vi "nanocal -- nuclear schottky fit V4.vi"() -> ()   [LabVIEW 2020] (continued)
  w19 = string[] ["T", "B", "theta", "side", "zeta", "tau1", "tauS", "tauN", "tauC", "kappa0"]  # names in latin
  w17 = string[] ["T", "B", "θ", "side", "ζ", "τ1", "τS", "τN", "τC", "κ0"]  # names greek
  w21 = map{T5, map{T11, string}} {}  # Size: 0
  w20 = T5[] [enum."T (K)", enum."B (T)", enum."θ (deg)", enum."side (S|R)", enum."ζ", enum."τ1", enum."τS", enum."τN", enum."τC", enum."κ0"] items=["ζ", "τ1", "τS", "τN", "τC", "κ0", "m1", "m2", "m3", "T (K)", "B (T)", "θ (deg)", "side (S|R)", "change (B|T)"]
  w27 = dbl[] []
  (unwired) u32[] [10967551, 1239551, 2785279, 16734592, 16755712, 8795, 8285330, 9272482, 9204890]
  w23 = T5[] [enum."ζ", enum."τ1", enum."τS", enum."τN", enum."τC", enum."κ0"] items=["ζ", "τ1", "τS", "τN", "τC", "κ0", "m1", "m2", "m3", "T (K)", "B (T)", "θ (deg)", "side (S|R)", "change (B|T)"]
  w33 = map{T5, i32} {}  # Size: 0
  w28 = T5[] [enum."ζ", enum."τ1", enum."τS", enum."τN", enum."τC", enum."κ0", enum."m1", enum."m2", enum."m3"] items=["ζ", "τ1", "τS", "τN", "τC", "κ0", "m1", "m2", "m3", "T (K)", "B (T)", "θ (deg)", "side (S|R)", "change (B|T)"]
  w34 = FALSE ("newton pause")
  w36 = map{T5, dbl} {}  # Size: 0
  w37 = 0.0 ("new X")
  w51 = "void"  # interface
  w53 = "void"  # action
  # "init file meta semantics -- external (file) part of the file key"
  # "cursor indices and plot colors"
  # "selector name semantics"
  # "init side semantics -- internal part of the file key"
  n1 = for {
    shift-right: [w62] -> w10
    shift-left: w13 -> [w63]
    tunnel: string[] ["_ref_", "_sam_"] -> [w59] mode=indexing
    tunnel: i32[] [4000, 8000] -> [w56] mode=indexing
    tunnel: w9 -> [w55] mode=indexing
    shift-right: [w60] -> w7
    shift-left: w8 -> [w61]
    shift-right: [w57] -> w5
    shift-left: w6 -> [w58]
    n2 = Insert Into Map(map in=w58, key=w56, value=w55) -> (map out=w57:map{i32, T14})  [unwired: 2 out]
    n3 = Insert Into Map(map in=w61, key=w55, value=w59) -> (map out=w60:map{T14, string})  [unwired: 2 out]
    n4 = Insert Into Map(map in=w63, key=w55, value=w56) -> (map out=w62:map{T14, i32})  [unwired: 2 out]
  }
  "side map from NUM" <- w5
  "side map to STR" <- w7
  "side map to NUM" <- w10
  n5 = for {
    shift-right: [w66] -> w4
    shift-left: w3 -> [w67]
    tunnel: w2 -> [w65] mode=indexing
    tunnel: w1 -> [w64] mode=indexing
    n6 = Insert Into Map(map in=w67, key=w65, value=w64) -> (map out=w66:map{T5, T15})  [unwired: 2 out]
  }
  "data file parameters map" <- w4
  n7 = for {
    shift-right: [w70] -> w31
    shift-left: w33 -> [w71]
    tunnel: w28 -> [w69] mode=indexing
    tunnel: i32[] [0, 1, 2, 3, 4, 5, 6, 7, 8] -> [w68] mode=indexing
    n8 = Insert Into Map(map in=w71, key=w69, value=w68) -> (map out=w70:map{T5, i32})  [unwired: 2 out]
  }
  n9 = for {
    shift-right: [w86] -> w15
    shift-left: w21 -> [w87]
    tunnel: w19 -> [w77] mode=indexing
    tunnel: w20 -> [w85] mode=indexing
    tunnel: w18 -> [w75]
    tunnel: w17 -> [w76] mode=indexing
    tunnel: w16 -> [w78] mode=indexing
    tunnel: w14 -> [w74] mode=indexing
    n10 = Insert Into Map(map in=w75, key=nameformattingitem."prec", value=w74) -> (map out=w73:map{T11, string})  [unwired: 2 out]
    n11 = Insert Into Map(map in=w73, key=nameformattingitem."name", value=w76) -> (map out=w84:map{T11, string})  [unwired: 2 out]
    n12 = Insert Into Map(map in=w84, key=nameformattingitem."nameL" ("name formatting item"), value=w77) -> (map out=w83:map{T11, string})  [unwired: 2 out]
    n13 = Insert Into Map(map in=w83, key=nameformattingitem."units" ("name formatting item"), value=w78) -> (map out=w82:map{T11, string})  [unwired: 2 out]
    n14 = Insert Into Map(map in=w87, key=w85, value=w82) -> (map out=w86:map{T5, map{T11, string}})  [unwired: 2 out]
  }
  "new selector names" <- w15
  n15 = local write "cursor index map"(w31) -> ()
  n16 = local write "newton action"(3-lorentzian-heat-response_action."onlygrads" ("newton action")) -> ()
  n17 = Bundle(w27, w27) -> (w26:cluster{dbl[], dbl[]})  [unwired: 1 in]
  n18 = Initialize Array(w26, 5 ("dimension size")) -> (→"Plot: goodness vs parameter":cluster{dbl[], dbl[]}[])
  n19 = control-ref of="Plot: sweep window"() -> (w43:refnum<vi>)
  n20 = Bundle By Name(cluster=T2 {"left"=0.0, "right "=0.0, "center"=0.0, "window"=0.0, "cursors"=[], "relative"=0, "absolute"=0, "fixed vertical offset"=0.0, "vertical offset"=0.0, "skew"=0.0, "default window frac"=0.0, "kind"=enum."symmetric", "skew.left"=0.0, "skew.right"=0.0, "Plot ref"=refnum, "wing order"=enum."forw"} ("cursor bracket: All, data window"), "Plot ref"=w43, "cursors"=i32[] [0, 1, 2], "fixed vertical offset"=0.0, "default window frac"=0.3 ("fixed vertical offset"), "kind"=enum16{"symmetric", "skewed", "fancy"}."symmetric") -> (w46:T2)
  n21 = local write "what"(cluster{"scaling":dbl, "what":T5}[] [{"scaling"=1.0, "what"=enum."ζ"}, {"scaling"=1.0, "what"=enum."τ1"}, {"scaling"=1.0, "what"=enum."τS"}, {"scaling"=1.0, "what"=enum."τN"}, {"scaling"=1.0, "what"=enum."τC"}, {"scaling"=1.0, "what"=enum."κ0"}]) -> ()
  n22 = control-ref of="cursor window"() -> (w42:refnum<vi>)
  n23 = Create User Event(user event datatype=w53) -> (user event=w41:refnum<user-event>)  [unwired: 1 in, 1 out]
  n24 = call "cursor window logic V3.vi"("cursor window action"=cursor_window_action."init", "cursor window in"=w42, "cursor window init"=w46) -> ()  [unwired: 7 in, 2 out]
  n25 = register-events(w41) -> (reference out=w54:refnum<event-registration>)  [unwired: 2 in, 1 out]
  n26 = Create User Event(user event datatype=w51) -> (user event=w29:refnum<user-event>)  [unwired: 1 in, 1 out]
  n27 = local write "parameter"(w23) -> ()
  n28 = register-events(w29) -> (reference out=w52:refnum<event-registration>)  [unwired: 2 in, 1 out]
  n29 = control-ref of="Plot: sweep window"() -> (w38:refnum<vi>)
  n30 = while "actions" {
    tunnel: w54 -> [w92]
    tunnel: w41 -> [w91]
    tunnel: w29 -> [w89]
    tunnel: w23 -> [w88]
    stop <- w90 stop-if-true
    n31 = event shown="[0] <action>: User Event" {
      selector: w92 -> [_]
      dyn-events: _ -> [_]
      timeout: _ -> [_]
      tunnel: w91 -> [w96]
      tunnel: [w95] -> w90
      tunnel: w89 -> [w94]
      tunnel: w88 -> [w93]
      event User Event {
        n32 = event-data() -> ("action"=w97:string)  [unwired: 1 in]
        n33 = case shown="\"action: constrained filenames select\"" w97 {
          tunnel: w96 -> [w98 _ _ w350 w457 w475 w495 _ w651 _ w769 _ _ w904 _ w981 w1020 _ w1077 _ _]
          tunnel: [_ _ _ _ _ _ _ _ _ _ _ _ _ _ _ _ _ TRUE _ _ _] -> w95
          tunnel: w94 -> [_ _ _ w349 _ _ _ _ _ _ _ _ _ _ _ _ _ _ _ _ _]
          tunnel: w93 -> [w100 w177 w233 _ _ _ _ _ _ _ _ _ w816 _ _ _ _ _ _ _ _]
          frame "action: new sweep" {
            (unwired) 3-lorentzian-heat-response_action."onlygrads" ("action")
            w106 = T5[] [enum."m1", enum."m2", enum."m3"] items=["ζ", "τ1", "τS", "τN", "τC", "κ0", "m1", "m2", "m3", "T (K)", "B (T)", "θ (deg)", "side (S|R)", "change (B|T)"]
            w112 = T5[] [enum."T (K)", enum."B (T)", enum."θ (deg)"] items=["ζ", "τ1", "τS", "τN", "τC", "κ0", "m1", "m2", "m3", "T (K)", "B (T)", "θ (deg)", "side (S|R)", "change (B|T)"]
            w149 = 6.283185307179586
            n34 = Generate User Event(user event=w98, event data cluster="action: reset colors" ("event data")) -> ()  [unwired: 2 in, 2 out]
            n35 = local read "T1"() -> (w135:dbl)
            n36 = call "nanocal -- publish -- freq scan V2.vi"("publisher action"=publisher_action."get") -> ("dz/dω out (V)"=w150:cdb[], "z out (V)"=w145:cdb[], "ω out (Hz)"=w152:dbl[])  [unwired: 8 in]
            n37 = local read "τS"() -> (w134:dbl)
            n38 = local read "τN"() -> (w133:dbl)
            n39 = local read "τC"() -> (w132:dbl)
            n40 = local read "κ0"() -> (w131:dbl)
            n41 = local read "ζ"() -> (w136:dbl)
            n42 = Divide(x=w150, y=w149) -> (x/y=w147:cdb[])
            n43 = Multiply(x=w152, y=w149) -> (x*y=w144:dbl[])
            n44 = Build Array (concatenate)(w100, w106) -> (w105:T5[])
            n45 = Build Array(w136, w135, w134, w133, w132, w131) -> (w118:dbl[])
            n46 = local read "newton action"() -> (w101:T9)
            n47 = for {
              shift-right: [w163] -> w104
              shift-left: map{T5, dbl} {} ("Map IN") -> [w164]
              tunnel: w105 -> [w161] mode=indexing
              tunnel: w118 -> [w162] mode=indexing
              tunnel: [w161] -> w107 mode=indexing
              n48 = Insert Into Map(map in=w164, key=w161, value=w162) -> (map out=w163:map{T5, dbl})  [unwired: 2 out]
            }
            n49 = local read "weighting"() -> (w146:T8)
            n50 = call "nanocal -- nuclear schottky goodness V5.vi"("action"=w101, "parameters IN"=w104, "weighting strategy"=w146, "dz/dω IN (V)"=w147, "Voltage IN (V)"=w145, "ω (rad/sec)"=w144) -> ("R norm"=w143:dbl, "G"=w142:dbl, "R(ω) out"=w141:cdb[], "dG / d log α   OUT"=w103:map{T5, dbl})  [unwired: 2 in]
            n51 = for {
              tunnel: w100 -> [w155] mode=indexing
              shift-right: [w156] -> _
              shift-left: w103 -> [w156]
              tunnel: [w154] -> w102 mode=indexing
              n52 = Look In Map(map=w156, key=w155) -> (value=w154:dbl)  [unwired: 1 in, 1 out]
            }
            "logarithmic derivatives" <- w102
            n53 = Divide(x=w142, y=w143) -> (x/y=→"goodness":dbl)
            n54 = local read "θ (deg)"() -> (w114:dbl)
            n55 = local read "B (T)"() -> (w115:dbl)
            n56 = local read "T (K)"() -> (w116:dbl)
            n57 = call "3-lorentzian-heat-response -- V4.vi"("action"=3-lorentzian-heat-response_action."calc m1m2m3", "Map IN"=w104) -> ("Map OUT"=w113:map{T5, dbl})  [unwired: 7 in, 2 out]
            n58 = Build Array(w116, w115, w114) -> (w111:dbl[])
            n59 = local read "cursor x selector"() -> (w140:map{T5, dbl})
            n60 = local read "X selector"() -> (w139:T5)
            n61 = local read "cursor index map"() -> (w120:map{T5, i32})
            n62 = for {
              shift-right: [w159] -> w110
              shift-left: w113 -> [w160]
              tunnel: w112 -> [w158] mode=indexing
              tunnel: w111 -> [w157] mode=indexing
              n63 = Insert Into Map(map in=w160, key=w158, value=w157) -> (map out=w159:map{T5, dbl})  [unwired: 2 out]
            }
            n64 = local read "T (K)"() -> (w138:dbl)
            n65 = control-ref of="Plot:  colors"() -> (w151:refnum<vi>)
            n66 = control-ref of="Plot: sweep window"() -> (w130:refnum<vi>)
            n67 = Complex To Re/Im(x + iy=w145) -> (x=w129:dbl[], y=w128:dbl[])
            n68 = Look In Map(map=w140, key=w139, default value=w138) -> (value=w137:dbl)  [unwired: 1 out]
            n69 = call "replace plot - plot ref - V2.vi"("Plot ref in"=w130, "Array X IN"=w129, "Array Y IN"=w128, "plot index"=enum16{"data R(ω)", "fit R(ω)"}."data R(ω)" ("Plost: sweep window"), "cursor action"=cursor_action."write") -> ("Plot ref out"=w127:refnum<vi>)  [unwired: 11 in, 3 out]
            n70 = for {
              tunnel: w137 -> [w172]
              tunnel: w151 -> [w171]
              tunnel: w107 -> [w167] mode=indexing
              tunnel: w120 -> [w169]
              shift-right: [w166] -> _
              shift-left: w113 -> [w166]
              n71 = Look In Map(map=w166, key=w167) -> (value=w165:dbl)  [unwired: 1 in, 1 out]
              n72 = Look In Map(map=w169, key=w167) -> (value=w168:i32)  [unwired: 1 in, 1 out]
              n73 = call "replace cursor - plot ref - V2.vi"("Plot ref in"=w171, "new X"=w172, "new  Y"=w165, "cursor index"=w168, "cursor action"=cursor_action."write") -> ()  [unwired: 11 in, 4 out]
            }
            n74 = call "string parse mathematica assosiated array.vi"("derivative"=mathematica_string_map_action."create string", "Map IN"=w110) -> ("String OUT"=w108:string)  [unwired: 8 in, 1 out]
            n75 = Complex To Re/Im(x + iy=w141) -> (x=w125:dbl[], y=w124:dbl[])
            n76 = local write "String"(w108) -> ()
            n77 = call "replace plot - plot ref - V2.vi"("Plot ref in"=w127, "Array X IN"=w125, "Array Y IN"=w124, "plot index"=enum16{"data R(ω)", "fit R(ω)"}."fit R(ω)" ("Plost: sweep window"), "cursor action"=cursor_action."write") -> ()  [unwired: 11 in, 4 out]
          }
          frame "action: replot circles" {
            w205 = 6.283185307179586
            n78 = call "nanocal -- publish -- freq scan V2.vi"("publisher action"=publisher_action."get") -> ("dz/dω out (V)"=w206:cdb[], "z out (V)"=w202:cdb[], "ω out (Hz)"=w207:dbl[])  [unwired: 8 in]
            n79 = local read "T1"() -> (w196:dbl)
            n80 = local read "τS"() -> (w195:dbl)
            n81 = local read "κ0"() -> (w192:dbl)
            n82 = local read "τN"() -> (w194:dbl)
            n83 = local read "τC"() -> (w193:dbl)
            n84 = local read "ζ"() -> (w197:dbl)
            n85 = Divide(x=w206, y=w205) -> (x/y=w204:cdb[])
            n86 = Multiply(x=w207, y=w205) -> (x*y=w201:dbl[])
            n87 = Build Array(w197, w196, w195, w194, w193, w192) -> (w178:dbl[])
            n88 = for {
              shift-right: [w214] -> w176
              shift-left: map{T5, dbl} {} ("Map IN") -> [w215]
              tunnel: w177 -> [w213] mode=indexing
              tunnel: [w212] -> _ mode=indexing
              tunnel: [w213] -> w174 mode=indexing
              tunnel: w178 -> [w212] mode=indexing
              n89 = Insert Into Map(map in=w215, key=w213, value=w212) -> (map out=w214:map{T5, dbl})  [unwired: 2 out]
            }
            n90 = local read "weighting"() -> (w203:T8)
            n91 = call "nanocal -- nuclear schottky goodness V5.vi"("action"=3-lorentzian-heat-response_action."onlygrads", "parameters IN"=w176, "weighting strategy"=w203, "dz/dω IN (V)"=w204, "Voltage IN (V)"=w202, "ω (rad/sec)"=w201) -> ("R norm"=w200:dbl, "G"=w199:dbl, "R(ω) out"=w198:cdb[], "dG / d log α   OUT"=w175:map{T5, dbl})  [unwired: 2 in]
            n92 = control-ref of="Plot: sweep window"() -> (w188:refnum<vi>)
            n93 = Divide(x=w199, y=w200) -> (x/y=w191:dbl)
            n94 = for {
              tunnel: w174 -> [w210] mode=indexing
              shift-right: [w211] -> _
              shift-left: w175 -> [w211]
              tunnel: [w209] -> w173 mode=indexing
              n95 = Look In Map(map=w211, key=w210) -> (value=w209:dbl)  [unwired: 1 in, 1 out]
            }
            n96 = Complex To Re/Im(x + iy=w202) -> (x=w186:dbl[], y=w185:dbl[])
            n97 = local write "goodness"(w191) -> ()
            n98 = call "replace plot - plot ref - V2.vi"("Plot ref in"=w188, "Array X IN"=w186, "Array Y IN"=w185, "plot index"=enum16{"data R(ω)", "fit R(ω)"}."data R(ω)" ("Plost: sweep window"), "cursor action"=cursor_action."write") -> ("Plot ref out"=w187:refnum<vi>)  [unwired: 11 in, 3 out]
            n99 = Complex To Re/Im(x + iy=w198) -> (x=w184:dbl[], y=w183:dbl[])
            n100 = local write "logarithmic derivatives"(w173) -> ()
            n101 = call "replace plot - plot ref - V2.vi"("Plot ref in"=w187, "Array X IN"=w184, "Array Y IN"=w183, "plot index"=enum16{"data R(ω)", "fit R(ω)"}."fit R(ω)" ("Plost: sweep window"), "cursor action"=cursor_action."write") -> ()  [unwired: 11 in, 4 out]
          }
          frame "action: plot landscape" {
            w225 = array_action."generate log range" ("action")
            w247 = 6.283185307179586
            n102 = property on="range one" class="Slide (strict)"() -> ("Scale.Range"=w237:T29)  [unwired: 2 in, 2 out]
            n103 = property on="range two" class="Slide (strict)"() -> ("Scale.Range"=w236:T29)  [unwired: 2 in, 2 out]
            n104 = Unbundle By Name(w237) -> ("Maximum"=w228:dbl, "Minimum"=w227:dbl)
            n105 = Unbundle By Name(w236) -> ("Maximum"=w230:dbl, "Minimum"=w229:dbl)
            n106 = local read "ζ"() -> (w243:dbl)
            n107 = local read "T1"() -> (w242:dbl)
            n108 = local read "τS"() -> (w241:dbl)
            n109 = local read "τN"() -> (w240:dbl)
            n110 = local read "τC"() -> (w239:dbl)
            n111 = local read "κ0"() -> (w238:dbl)
            n112 = call "nanocal -- publish -- freq scan V2.vi"("publisher action"=publisher_action."get") -> ("dz/dω out (V)"=w248:cdb[], "z out (V)"=w245:cdb[], "ω out (Hz)"=w249:dbl[])  [unwired: 8 in]
            n113 = local read "cursor index map"() -> (w219:map{T5, i32})
            n114 = Build Array(w243, w242, w241, w240, w239, w238) -> (w224:dbl[])
            n115 = call "array -- generate range -- V5.vi"("action"=w225, "ω points"="# points", "ω from"=w227, "ω to"=w228) -> ("ω out"=w226:dbl[])  [unwired: 7 in]
            n116 = call "array -- generate range -- V5.vi"("action"=w225, "ω points"="# points", "ω from"=w229, "ω to"=w230) -> ("ω out"=w231:dbl[])  [unwired: 7 in]
            n117 = local read "color Map"() -> (w220:map{T5, u32})
            n118 = Divide(x=w248, y=w247) -> (x/y=w246:cdb[])
            n119 = Multiply(x=w249, y=w247) -> (x*y=w244:dbl[])
            n120 = for {
              shift-right: [w340] -> w232
              shift-left: map{T5, dbl} {} ("Map IN") -> [w341]
              tunnel: w233 -> [w339] mode=indexing
              tunnel: w224 -> [w338] mode=indexing
              n121 = Insert Into Map(map in=w341, key=w339, value=w338) -> (map out=w340:map{T5, dbl})  [unwired: 2 out]
            }
            n122 = Look In Map(map=w220, key="two") -> (value=w222:u32)  [unwired: 1 in, 1 out]
            n123 = Look In Map(map=w220, key="one") -> (value=w221:u32)  [unwired: 1 in, 1 out]
            n124 = property on="range one" class="Slide (strict)"("Fill Color"=w221) -> ()  [unwired: 2 in, 2 out]
            n125 = Build Array("one", "two") -> (w218:T5[])
            n126 = property on="range two" class="Slide (strict)"("Fill Color"=w222) -> ()  [unwired: 2 in, 2 out]
            n127 = case shown="\"2d plots \"" "what" {
              tunnel: w246 -> [w259 w302]
              tunnel: w245 -> [w258 w301]
              tunnel: w244 -> [w257 w300]
              tunnel: w232 -> [w256 w299]
              tunnel: "one" -> [_ w298]
              tunnel: w231 -> [_ w297]
              tunnel: w226 -> [w255 w296]
              tunnel: "two" -> [_ w295]
              tunnel: w220 -> [w254 _]
              tunnel: w219 -> [w253 _]
              tunnel: w218 -> [w251 _]
              frame "1d plots", Default {
                n128 = control-ref of="Plot: goodness vs parameter"() -> (w252:refnum<vi>)
                n129 = for {
                  tunnel: w259 -> [w278]
                  tunnel: w258 -> [w277]
                  tunnel: w257 -> [w276]
                  tunnel: w256 -> [w263]
                  tunnel: w255 -> [w272]
                  tunnel: w251 -> [w262] mode=indexing
                  tunnel: w254 -> [w269]
                  tunnel: w253 -> [w268]
                  tunnel: w252 -> [w260]
                  n130 = for {
                    tunnel: w278 -> [w283]
                    tunnel: w277 -> [w285]
                    tunnel: w276 -> [w284]
                    tunnel: w272 -> [w280] mode=indexing
                    tunnel: [w288] -> w274 mode=indexing
                    tunnel: [w280] -> w273 mode=indexing
                    tunnel: w263 -> [w281]
                    tunnel: w262 -> [w282]
                    n131 = Insert Into Map(map in=w281, key=w282, value=w280) -> (map out=w279:map{T5, dbl})  [unwired: 2 out]
                    n132 = local read "weighting"() -> (w287:T8)
                    n133 = call "nanocal -- nuclear schottky goodness V5.vi"("action"=3-lorentzian-heat-response_action."onlygrads", "parameters IN"=w279, "weighting strategy"=w287, "dz/dω IN (V)"=w283, "Voltage IN (V)"=w285, "ω (rad/sec)"=w284) -> ("R norm"=w290:dbl, "G"=w289:dbl)  [unwired: 2 in, 2 out]
                    n134 = Divide(x=w289, y=w290) -> (x/y=w288:dbl)
                  }
                  n135 = Look In Map(map=w263, key=w262) -> (value=w261:dbl)  [unwired: 1 in, 1 out]
                  n136 = Look In Map(map=w269, key=w262) -> (value=w264:u32)  [unwired: 1 in, 1 out]
                  n137 = Look In Map(map=w268, key=w262) -> (value=w266:i32)  [unwired: 1 in, 1 out]
                  n138 = call "replace plot - plot ref - V2.vi"("Plot ref in"=w260, "Array X IN"=w273, "Array Y IN"=w274, "plot index"=w266, "cursor action"=cursor_action."write") -> ("Plot ref out"=w271:refnum<vi>)  [unwired: 11 in, 3 out]
                  n139 = call "replace cursor - plot ref - V2.vi"("Plot ref in"=w260, "new X"=w261, "cursor index"=w266, "cursor action"=cursor_action."write", "Color Box"=w264, "cursor state"=cursor_sate."colored") -> ()  [unwired: 10 in, 4 out]
                  n140 = call "replace plot - plot ref - V2.vi"("Plot ref in"=w271, "plot index"=w266, "cursor action"=cursor_action."set plot color", "Color Box"=w264) -> ()  [unwired: 12 in, 4 out]
                }
              }
              frame "2d plots " {
                n141 = for {
                  tunnel: w302 -> [w312]
                  tunnel: w301 -> [w311]
                  tunnel: w300 -> [w310]
                  tunnel: w299 -> [w309]
                  tunnel: w298 -> [w308]
                  tunnel: w297 -> [w307] mode=indexing
                  tunnel: w296 -> [w306]
                  tunnel: w295 -> [w305]
                  shift-right: [w303] -> w292
                  shift-left: "{ " -> [w304]
                  n142 = for {
                    tunnel: w312 -> [w331]
                    tunnel: w311 -> [w333]
                    tunnel: w310 -> [w332]
                    tunnel: w306 -> [w314] mode=indexing
                    tunnel: w307 -> [w313]
                    tunnel: w309 -> [w329]
                    tunnel: w308 -> [w330]
                    tunnel: w305 -> [w328]
                    shift-right: [w324] -> w303
                    shift-left: w304 -> [w325]
                    w317 = " ,     "
                    w323 = i16 12 ("precision (6)")
                    n143 = Insert Into Map(map in=w329, key=w330, value=w314) -> (map out=w326:map{T5, dbl})  [unwired: 2 out]
                    n144 = Insert Into Map(map in=w326, key=w328, value=w313) -> (map out=w327:map{T5, dbl})  [unwired: 2 out]
                    n145 = local read "weighting"() -> (w335:T8)
                    n146 = Number To Fractional String(number=w314, precision (6)=w323) -> (F-format string=w321:string)  [unwired: 2 in]
                    n147 = call "nanocal -- nuclear schottky goodness V5.vi"("action"=3-lorentzian-heat-response_action."onlygrads", "parameters IN"=w327, "weighting strategy"=w335, "dz/dω IN (V)"=w331, "Voltage IN (V)"=w333, "ω (rad/sec)"=w332) -> ("R norm"=w337:dbl, "G"=w336:dbl)  [unwired: 2 in, 2 out]
                    n148 = Number To Fractional String(number=w313, precision (6)=w323) -> (F-format string=w320:string)  [unwired: 2 in]
                    n149 = Divide(x=w336, y=w337) -> (x/y=w322:dbl)
                    n150 = Number To Fractional String(number=w322, precision (6)=w323) -> (F-format string=w319:string)  [unwired: 2 in]
                    n151 = Concatenate Strings(w325, "{    ", w321, w317, w320, w317, w319, " } , ", "\r") -> (w324:string)
                  }
                }
                n152 = Concatenate Strings(w292, " }   ") -> (→"2dplots":string)
              }
            }
          }
          frame "action: gradient step" {
            w346 = 6.283185307179586
            w351 = FALSE ("newton pause")
            n153 = call "nanocal -- publish -- freq scan V2.vi"("publisher action"=publisher_action."get") -> ("dz/dω out (V)"=w348:cdb[], "z out (V)"=w343:cdb[], "ω out (Hz)"=w347:dbl[])  [unwired: 8 in]
            n154 = local write "newton pause"(w351) -> ()
            n155 = Generate User Event(user event=w350, event data cluster="action: new sweep" ("event data")) -> ()  [unwired: 2 in, 2 out]
            n156 = Divide(x=w348, y=w346) -> (x/y=w344:cdb[])
            n157 = Multiply(x=w347, y=w346) -> (x*y=w342:dbl[])
            n158 = for {
              N: "# steps" -> [_]
              tunnel: [TRUE ("newton pause")] -> w352
              tunnel: w351 -> [_]
              shift-right: [w388] -> _
              shift-left: w349 -> [w388]
              tunnel: w344 -> [w371]
              tunnel: w343 -> [w370]
              tunnel: w342 -> [w369]
              stop <- w396 stop-if-true
              (unwired) 3-lorentzian-parameters."κ0" ("Plost: sweep window")
              (unwired) 3-lorentzian-parameters."τC" ("Plost: sweep window")
              (unwired) 3-lorentzian-parameters."τN" ("Plost: sweep window")
              (unwired) 3-lorentzian-parameters."τS" ("Plost: sweep window")
              (unwired) 3-lorentzian-parameters."τ1" ("Plost: sweep window")
              (unwired) 3-lorentzian-parameters."ζ" ("Plost: sweep window")
              w366 = T5[] [enum."ζ", enum."τ1", enum."τS", enum."τN", enum."τC", enum."κ0"] items=["ζ", "τ1", "τS", "τN", "τC", "κ0", "m1", "m2", "m3", "T (K)", "B (T)", "θ (deg)", "side (S|R)", "change (B|T)"]
              n159 = local read "newton pause"() -> (w396:bool)
              n160 = local read "T1"() -> (w401:dbl)
              n161 = local read "τS"() -> (w400:dbl)
              n162 = local read "τN"() -> (w399:dbl)
              n163 = local read "τC"() -> (w398:dbl)
              n164 = local read "κ0"() -> (w397:dbl)
              n165 = local read "ζ"() -> (w402:dbl)
              n166 = Build Array(w402, w401, w400, w399, w398, w397) -> (w373:dbl[])
              n167 = for {
                shift-right: [w425] -> w372
                shift-left: map{T5, dbl} {} ("Map IN") -> [w426]
                tunnel: w366 -> [w423] mode=indexing
                tunnel: w373 -> [w424] mode=indexing
                tunnel: [w423] -> w365 mode=indexing
                n168 = Insert Into Map(map in=w426, key=w423, value=w424) -> (map out=w425:map{T5, dbl})  [unwired: 2 out]
              }
              n169 = local read "newton action"() -> (w357:T9)
              n170 = local read "factor"() -> (w355:dbl)
              n171 = local read "weighting"() -> (w356:T8)
              n172 = local read "what"() -> (w360:cluster{"scaling":dbl, "what":T5}[])
              n173 = call "nanocal -- nuclear schottky goodness V5.vi"("action"=w357, "parameters IN"=w372, "weighting strategy"=w356, "dz/dω IN (V)"=w371, "Voltage IN (V)"=w370, "ω (rad/sec)"=w369) -> ("R norm"=w363:dbl, "G"=w364:dbl, "R(ω) out"=w368:cdb[], "dG / d log α   OUT"=w367:map{T5, dbl})  [unwired: 2 in]
              n174 = Complex To Re/Im(x + iy=w368) -> (x=w385:dbl[], y=w384:dbl[])
              n175 = control-ref of="Plot: sweep window"() -> (w387:refnum<vi>)
              n176 = call "3-lorentzian-heat-response -- V4.vi"("action"=3-lorentzian-heat-response_action."calc m1m2m3", "Map IN"=w372) -> ("Map OUT"=w376:map{T5, dbl})  [unwired: 7 in, 2 out]
              n177 = for {
                tunnel: w365 -> [w421] mode=indexing
                shift-right: [w422] -> _
                shift-left: w367 -> [w422]
                tunnel: [w417] -> w361 mode=indexing
                tunnel: w360 -> [w420] mode=indexing
                tunnel: w355 -> [w416]
                tunnel: [w415] -> w359 mode=indexing
                n178 = Unbundle By Name(w420) -> ("scaling"=w418:dbl)
                n179 = Look In Map(map=w422, key=w421) -> (value=w417:dbl)  [unwired: 1 in, 1 out]
                n180 = Compound Arithmetic op=MULTIPLY(w418, w416, -1.0 ("index"), w417) -> (w415:dbl)
              }
              n181 = local read "cursor x selector"() -> (w381:map{T5, dbl})
              n182 = local read "X selector"() -> (w380:T5)
              n183 = local read "cursor index map"() -> (w377:map{T5, i32})
              n184 = call "replace plot - plot ref - V2.vi"("Plot ref in"=w387, "Array X IN"=w385, "Array Y IN"=w384, "plot index"=enum16{"data R(ω)", "fit R(ω)"}."fit R(ω)" ("Plost: sweep window"), "cursor action"=cursor_action."write") -> ()  [unwired: 11 in, 4 out]
              n185 = local read "T (K)"() -> (w379:dbl)
              n186 = control-ref of="Plot:  colors"() -> (w382:refnum<vi>)
              n187 = Look In Map(map=w381, key=w380, default value=w379) -> (value=w378:dbl)  [unwired: 1 out]
              n188 = Exponential(1:w359) -> (0:w358:dbl[])
              n189 = for {
                tunnel: w378 -> [w434]
                tunnel: w382 -> [w433]
                tunnel: w366 -> [w429] mode=indexing
                tunnel: w377 -> [w431]
                shift-right: [w428] -> _
                shift-left: w376 -> [w428]
                n190 = Look In Map(map=w428, key=w429) -> (value=w427:dbl)  [unwired: 1 in, 1 out]
                n191 = Look In Map(map=w431, key=w429) -> (value=w430:i32)  [unwired: 1 in, 1 out]
                n192 = call "replace cursor - plot ref - V2.vi"("Plot ref in"=w433, "new X"=w434, "new  Y"=w427, "cursor index"=w430, "cursor action"=cursor_action."write") -> ()  [unwired: 11 in, 4 out]
              }
              n193 = Index Array(array=w358, index #1=3-lorentzian-parameters."ζ" ("Plost: sweep window"), index #2=3-lorentzian-parameters."τ1" ("Plost: sweep window"), index #3=3-lorentzian-parameters."τS" ("Plost: sweep window"), index #4=3-lorentzian-parameters."τN" ("Plost: sweep window"), index #5=3-lorentzian-parameters."τC" ("Plost: sweep window"), index #6=3-lorentzian-parameters."κ0" ("Plost: sweep window")) -> (element #1=w409:dbl, element #2=w408:dbl, element #3=w407:dbl, element #4=w406:dbl, element #5=w405:dbl, element #6=w403:dbl)
              n194 = Divide(x=w364, y=w363) -> (x/y=w362:dbl)
              n195 = local write "logarithmic derivatives"(w361) -> ()
              n196 = local write "goodness"(w362) -> ()
              n197 = Multiply(x=w409, y=w402) -> (x*y=w414:dbl)
              n198 = Multiply(x=w408, y=w401) -> (x*y=w413:dbl)
              n199 = Multiply(x=w407, y=w400) -> (x*y=w412:dbl)
              n200 = Multiply(x=w406, y=w399) -> (x*y=w411:dbl)
              n201 = Multiply(x=w405, y=w398) -> (x*y=w410:dbl)
              n202 = Multiply(x=w403, y=w397) -> (x*y=w404:dbl)
              n203 = local write "τN"(w411) -> ()
              n204 = local write "τC"(w410) -> ()
              n205 = local write "τS"(w412) -> ()
              n206 = local write "κ0"(w404) -> ()
              n207 = local write "T1"(w413) -> ()
              n208 = local write "ζ"(w414) -> ()
            }
            n209 = local write "newton pause"(w352) -> ()
          }
          frame "action: uco" {
            (unwired) 3-lorentzian-parameters."κ0" ("Plost: sweep window")
            n210 = local read "T1"() -> (w449:dbl)
            n211 = local read "τN"() -> (w447:dbl)
            n212 = local read "τC"() -> (w446:dbl)
            n213 = local read "κ0"() -> (w445:dbl)
            n214 = local read "τS"() -> (w448:dbl)
            n215 = local read "ζ"() -> (w450:dbl)
            n216 = Generate User Event(user event=w457, event data cluster="action: new sweep" ("event data")) -> ()  [unwired: 2 in, 2 out]
            n217 = call "3-lorentzian-parameters - manage.vi"("ζ"=w450, "T1"=w449, "τS"=w448, "τN"=w447, "τC"=w446, "κ0"=w445, "parameters"=3-lorentzian-parameters_--_action."to array") -> ("parameter array OUT"=w443:dbl[])  [unwired: 6 in, 6 out]
            n218 = Natural Logarithm(1:w443) -> (0:w455:dbl[])
            n219 = vi-ref "nanocal -- nuclear schottky goodness -- for UCO -- V3.vi"() -> (w456:refnum<vi>)
            n220 = call-poly <vilib>:"Unconstrained Optimization.vi"("function data"=T22 variant, "objective function"=w456, "start"=w455) -> ("f(minimum)"=w453:dbl, "minimum"=w454:dbl[])  [unwired: 5 in, 2 out]
            n221 = Exponential(1:w453) -> (0:w452:dbl)
            n222 = Exponential(1:w454) -> (0:w442:dbl[])
            n223 = call "3-lorentzian-parameters - manage.vi"("parameter array"=w442, "parameters"=3-lorentzian-parameters_--_action."to parameters") -> ("ζ OUT"=w441:dbl, "T1 OUT"=w440:dbl, "τS  OUT"=w439:dbl, "τN  OUT"=w438:dbl, "τC  OUT"=w437:dbl, "κ0  OUT"=w436:dbl)  [unwired: 11 in, 1 out]
            n224 = local write "goodness"(w452) -> ()
            n225 = local write "T1"(w440) -> ()
            n226 = local write "τN"(w438) -> ()
            n227 = local write "τC"(w437) -> ()
            n228 = local write "κ0"(w436) -> ()
            n229 = local write "τS"(w439) -> ()
            n230 = local write "ζ"(w441) -> ()
          }
          frame "action: parse string" {
            n231 = local read "String"() -> (w477:string)
            n232 = call "string parse mathematica assosiated array.vi"("derivative"=mathematica_string_map_action."parse string", "String in"=w477) -> ("Map OUT"=w471:map{T5, dbl})  [unwired: 8 in, 1 out]
            n233 = Generate User Event "action User Event"(user event=w475, event data cluster="action: update state of selectors" ("event data")) -> (user event out=w459:refnum<user-event>)  [unwired: 2 in, 1 out]
            n234 = Look In Map(map=w471, key=3-lorentzian-parameters."ζ" ("Plost: sweep window")) -> (value=w466:dbl)  [unwired: 1 in, 1 out]
            n235 = Look In Map(map=w471, key=3-lorentzian-parameters."τ1" ("Plost: sweep window")) -> (value=w465:dbl)  [unwired: 1 in, 1 out]
            n236 = Look In Map(map=w471, key=3-lorentzian-parameters."τS" ("Plost: sweep window")) -> (value=w464:dbl)  [unwired: 1 in, 1 out]
            n237 = Look In Map(map=w471, key=3-lorentzian-parameters."τN" ("Plost: sweep window")) -> (value=w463:dbl)  [unwired: 1 in, 1 out]
            n238 = Look In Map(map=w471, key=3-lorentzian-parameters."τC" ("Plost: sweep window")) -> (value=w462:dbl)  [unwired: 1 in, 1 out]
            n239 = Look In Map(map=w471, key=3-lorentzian-parameters."κ0" ("Plost: sweep window")) -> (value=w461:dbl)  [unwired: 1 in, 1 out]
            n240 = local write "ζ"(w466) -> ()
            n241 = local write "T1"(w465) -> ()
            n242 = local write "τS"(w464) -> ()
            n243 = local write "τN"(w463) -> ()
            n244 = local write "τC"(w462) -> ()
            n245 = local write "κ0"(w461) -> ()
            n246 = Generate User Event "action User Event"(user event=w459, event data cluster="action: replot colors" ("event data")) -> ()  [unwired: 2 in, 2 out]
          }
          frame "action: read mathematica string" {
            w478 = map{string, path} {}  # Size: 0
            w499 = map{T5, dbl} {}  # Size: 0
            w491 = set{dbl} {}  # Size: 0
            w501 = map{string, map{T5, dbl}} {}  # Size: 0
            w484 = map{string, string} {}  # Size: 0
            n247 = local read "file pattern"() -> (w481:string)
            n248 = local read "folder"() -> (w482:path)
            n249 = local read "data file parameters map"() -> (w487:map{T5, T15})
            n250 = call <vilib>:"Recursive File List.vi"("pattern"=w481, "Continue Recursing on Error? (F)"=TRUE, "Folder Path"=w482) -> ("All Files in Dir"=w479:path[])  [unwired: 4 in, 4 out]
            n251 = Generate User Event(user event=w495, event data cluster="action: update enums" ("event data")) -> ()  [unwired: 2 in, 2 out]
            n252 = local read "side map to NUM"() -> (w485:map{T14, i32})
            n253 = local read "side map to STR"() -> (w486:map{T14, string})
            n254 = call "string parse mathematica list assosiated array -- V2.vi"("derivative"=3-lorentzian-heat-response_action."parse string", "string IN"="string IN") -> ("Map OUT"=w502:map{string, map{T5, dbl}})  [unwired: 8 in, 1 out]
            n255 = for {
              tunnel: w479 -> [w505] mode=indexing
              shift-right: [w519] -> w488
              shift-left: w502 -> [w529]
              shift-right: [w516] -> w490
              shift-left: w484 -> [w528]
              shift-right: [w515] -> w489
              shift-left: w501 -> [w524]
              shift-right: [w526] -> w497
              shift-left: w491 -> [w518]
              shift-right: [w517] -> w498
              shift-left: w491 -> [w527]
              tunnel: w499 -> [w522]
              shift-right: [w512] -> w494
              shift-left: w491 -> [w525]
              shift-right: [w514] -> w493
              shift-left: w491 -> [w523]
              tunnel: w487 -> [w521]
              shift-right: [w513] -> w492
              shift-left: w491 -> [w520]
              tunnel: w485 -> [w510]
              tunnel: w486 -> [w509]
              shift-right: [w506] -> w483
              shift-left: w478 -> [w507]
              w508 = T14[] [enum."sam", enum."ref"] items=["sam", "ref"]
              n256 = Strip Path(path=w505) -> (name=w504:string)  [unwired: 1 out]
              n257 = call "filename-manage.vi"("filename-action"=filename-action."getIDStock", "file name IN"=w504) -> ("string OUT"=w511:string)  [unwired: 7 in, 2 out]
              n258 = for {
                tunnel: w521 -> [w555]
                tunnel: w504 -> [w532]
                tunnel: w511 -> [w544]
                shift-right: [w553] -> w519
                shift-left: w529 -> [w564]
                shift-right: [w559] -> w526
                shift-left: w518 -> [w552]
                shift-right: [w551] -> w517
                shift-left: w527 -> [w560]
                shift-right: [w545] -> w512
                shift-left: w525 -> [w558]
                shift-right: [w546] -> w514
                shift-left: w523 -> [w556]
                shift-right: [w547] -> w513
                shift-left: w520 -> [w554]
                shift-right: [w548] -> w515
                shift-left: w524 -> [w557]
                shift-right: [w549] -> w516
                shift-left: w528 -> [w563]
                tunnel: w510 -> [w537]
                tunnel: w522 -> [w542]
                tunnel: w509 -> [w539]
                tunnel: w508 -> [w536] mode=indexing
                shift-right: [w533] -> w506
                shift-left: w507 -> [w534]
                tunnel: w505 -> [w531]
                # "internal key"
                n259 = Look In Map(map=w537, key=w536) -> (value=w535:i32)  [unwired: 1 in, 1 out]
                n260 = Look In Map(map=w539, key=w536) -> (value=w538:string)  [unwired: 1 in, 1 out]
                n261 = Insert Into Map(map in=w542, key=3-lorentzian-parameters."side (S|R)", value=w535) -> (map out=w541:map{T5, dbl})  [unwired: 2 out]
                n262 = Concatenate Strings(w544, w538) -> (w543:string)
                n263 = for {
                  shift-right: [w570] -> w550
                  shift-left: w541 -> [w571]
                  tunnel: w555 -> [w569] mode=indexing
                  tunnel: w532 -> [w567]
                  n264 = Unbundle(w569) -> ("key"=w568:T5, "filename-action"=w566:T15)
                  n265 = call "filename-manage.vi"("filename-action"=w566, "file name IN"=w567) -> ("number OUT"=w565:dbl)  [unwired: 7 in, 2 out]
                  n266 = Insert Into Map(map in=w571, key=w568, value=w565) -> (map out=w570:map{T5, dbl})  [unwired: 2 out]
                }
                n267 = in-place {
                  in-place-border: [w613] -> w562
                  in-place-border: w550 -> [w612]
                  n268 = in-place-map #1(w564, w543) -> (w611:map{T5, dbl}, w613:bool)  [unwired: 1 in]
                  n269 = for {
                    tunnel: w612 -> [w619] mode=indexing
                    shift-right: [w617] -> w610
                    shift-left: w611 -> [w618]
                    n270 = Unbundle(w619) -> ("key"=w616:T5, "number OUT"=w615:dbl)
                    n271 = Insert Into Map(map in=w618, key=w616, value=w615) -> (map out=w617:map{T5, dbl})  [unwired: 2 out]
                  }
                  n272 = in-place-map #1(w610, LVMapReplaceAction."Modify Entry only if found" ("action")) -> (w553:map{string, map{T5, dbl}})  [unwired: 2 out]
                }
                n273 = Not(x=w562) -> (.not. x?=w561:bool)
                n274 = case shown="True" w561 {
                  tunnel: w563 -> [w579 w609]
                  tunnel: [w579 w608] -> w549
                  tunnel: w532 -> [_ w607]
                  tunnel: w543 -> [_ w581]
                  tunnel: w560 -> [w577 w606]
                  tunnel: [w577 w605] -> w551
                  tunnel: w552 -> [w578 w604]
                  tunnel: [w578 w603] -> w559
                  tunnel: [w575 w602] -> w545
                  tunnel: w558 -> [w575 w601]
                  tunnel: w550 -> [_ w586]
                  tunnel: w557 -> [w576 w600]
                  tunnel: [w576 w599] -> w548
                  tunnel: [w574 w598] -> w546
                  tunnel: w556 -> [w574 w597]
                  tunnel: [w573 w588] -> w547
                  tunnel: w554 -> [w573 w587]
                  tunnel: w534 -> [w572 w583]
                  tunnel: [w572 w582] -> w533
                  tunnel: w531 -> [_ w580]
                  frame False {
                  }
                  frame True {
                    n275 = Look In Map(map=w586, key=3-lorentzian-parameters."change (B|T)") -> (value=w589:dbl)  [unwired: 1 in, 1 out]
                    n276 = Look In Map(map=w586, key=3-lorentzian-parameters."side (S|R)") -> (value=w595:dbl)  [unwired: 1 in, 1 out]
                    n277 = Look In Map(map=w586, key=3-lorentzian-parameters."T (K)") -> (value=w593:dbl)  [unwired: 1 in, 1 out]
                    n278 = Look In Map(map=w586, key=3-lorentzian-parameters."B (T)") -> (value=w585:dbl)  [unwired: 1 in, 1 out]
                    n279 = Look In Map(map=w586, key=3-lorentzian-parameters."θ (deg)") -> (value=w584:dbl)  [unwired: 1 in, 1 out]
                    n280 = Insert Into Map(map in=w583, key=w581, value=w580) -> (map out=w582:map{string, path})  [unwired: 2 out]
                    n281 = Insert Into Set(10:w595, 11:w597) -> (3:w598:set{dbl})  [unwired: 1 out]
                    n282 = Insert Into Set(10:w593, 11:w601) -> (3:w602:set{dbl})  [unwired: 1 out]
                    n283 = Insert Into Set(10:w585, 11:w606) -> (3:w605:set{dbl})  [unwired: 1 out]
                    n284 = Insert Into Set(10:w584, 11:w604) -> (3:w603:set{dbl})  [unwired: 1 out]
                    n285 = Insert Into Map(map in=w600, key=w581, value=w586) -> (map out=w599:map{string, map{T5, dbl}})  [unwired: 2 out]
                    n286 = Insert Into Map(map in=w609, key=w581, value=w607) -> (map out=w608:map{string, string})  [unwired: 2 out]
                    n287 = Insert Into Set(10:w589, 11:w587) -> (3:w588:set{dbl})  [unwired: 1 out]
                  }
                }
              }
            }
            "Set of B's" <- w498
            "Set of θ's" <- w497
            "Set of T's" <- w494
            "Set of Sides" <- w493
            "Set of Change" <- w492
            "all short filenames" <- w490
            "temps&degs" <- w489
            "all full filenames" <- w483
            n288 = local write "mathematica thing"(w488) -> ()
          }
          frame "action: empty string from filelist" {
            n289 = local read "file pattern"() -> (w621:string)
            n290 = local read "folder"() -> (w622:path)
            n291 = call <vilib>:"Recursive File List.vi"("pattern"=w621, "Continue Recursing on Error? (F)"=TRUE, "Folder Path"=w622) -> ("All Files in Dir"=w620:path[])  [unwired: 4 in, 4 out]
            n292 = for {
              tunnel: [w628] -> w624 mode=concatenating
              tunnel: w620 -> [w633] mode=indexing
              w631 = T14[] [enum."ref", enum."sam"] items=["sam", "ref"]
              n293 = Strip Path(path=w633) -> (name=w632:string)  [unwired: 1 out]
              n294 = local read "side map to STR"() -> (w630:map{T14, string})
              n295 = call "filename-manage.vi"("filename-action"=filename-action."getIDStock", "file name IN"=w632) -> ("string OUT"=w629:string)  [unwired: 7 in, 2 out]
              n296 = for {
                tunnel: w631 -> [w638] mode=indexing
                tunnel: w630 -> [w639]
                tunnel: w629 -> [w637]
                tunnel: [w635] -> w628 mode=indexing
                n297 = Look In Map(map=w639, key=w638) -> (value=w636:string)  [unwired: 1 in, 1 out]
                n298 = Concatenate Strings(w637, w636) -> (w635:string)
              }
            }
            n299 = disable-structure shown="Disabled" {
              frame Disabled {
                n300 = List Folder() -> (filenames=w627:string[])  [unwired: 4 in, 3 out]
              }
              frame Enabled {
              }
            }
            n301 = call "string parse mathematica list assosiated array -- V2.vi"("derivative"=3-lorentzian-heat-response_action."create emty string", "array of IDs"=w624) -> ("string out"=w625:string)  [unwired: 8 in, 1 out]
            n302 = local write "string OUT"(w625) -> ()
          }
          frame "action: update enums" {
            w641 = map{string, string} {}  # Size: 0
            w646 = map{i32, dbl} {}  # Size: 0
            w650 = map{i32, dbl} {}  # Size: 0
            w656 = map{i32, dbl} {}  # Size: 0
            w663 = map{i32, string} {}  # Size: 0
            w662 = map{i32, dbl} {}  # Size: 0
            w661 = map{i32, dbl} {}  # Size: 0
            # "gives a key"
            n303 = local read "all short filenames"() -> (w642:map{string, string})
            n304 = local read "Set of T's"() -> (w655:set{dbl})
            n305 = local read "Set of Sides"() -> (w648:set{dbl})
            n306 = for {
              tunnel: w642 -> [w678] mode=indexing
              shift-right: [w676] -> w640
              shift-left: w641 -> [w677]
              n307 = Unbundle(w678) -> ("event data"=w674:string, "file pattern"=w675:string)
              n308 = Insert Into Map(map in=w677, key=w675, value=w674) -> (map out=w676:map{string, string})  [unwired: 2 out]
            }
            n309 = Generate User Event(user event=w651, event data cluster="action: update state of selectors" ("event data")) -> ()  [unwired: 2 in, 2 out]
            n310 = for {
              shift-right: [w693] -> w654
              shift-left: w656 -> [w694]
              tunnel: [w691] -> w653 mode=indexing
              tunnel: w655 -> [w690] mode=indexing
              i -> [w692]
